vi "FTW-CodeGen-GetGrowInfo.vi"(0 "State In":T2, 5 "XRef":refnum<vi>) -> (1 "Spacing Between Terminals":i32=8 format="%d pixels", 2 "Timing Terminal Height":i32=8 format="%d pixels", 3 "Timing Terminals":i32[](array[numeric]) format="%d pixels", 4 "Grow Info":T1, 6 "Current Height":i32=8 format="%d pixels", 8 "Width":i32=8 format="%d pixels", 10 "Terminal Height":i32=8 format="%d pixels", 13 "Bottom Banner Height":i32=8 format="%d pixels", 14 "Total Top Banner Height":i32=8 format="%d pixels")   [LabVIEW 2014, in "FTW-Dataflow-Synchronizer.xnode"]
uses:
  FTW-Dataflow-Synchronizer.xnode
  FTW-CodeGen-State.ctl
panel:
  # "Inputs"
  # "Outputs"
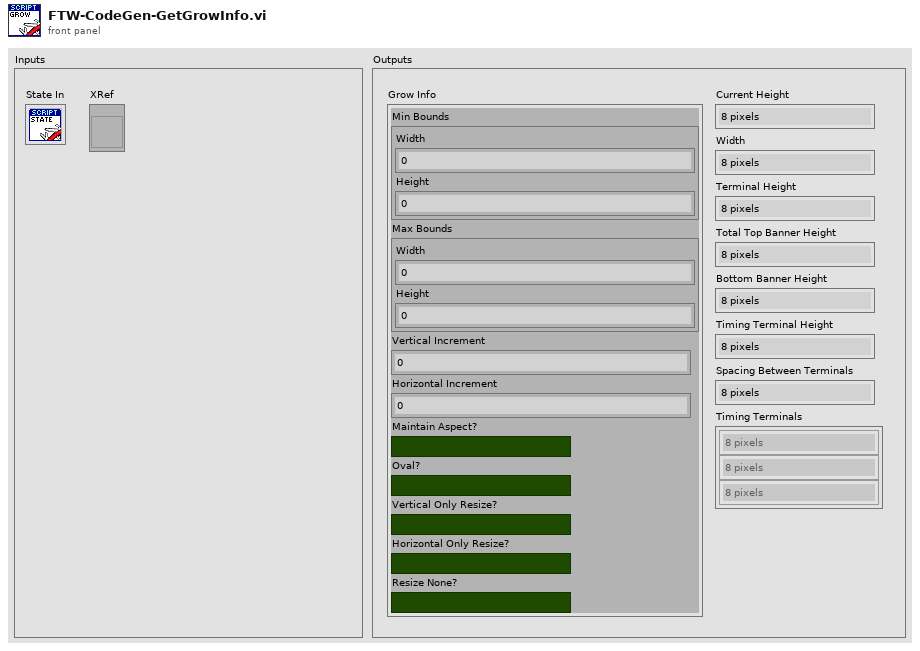
[diagram p1: front panel]
types:
  T1 = cluster{"Min Bounds":cluster{"Width":i32, "Height":i32}, "Max Bounds":cluster{"Width":i32, "Height":i32}, "Vertical Increment":i32, "Horizontal Increment":i32, "Maintain Aspect?":bool, "Oval?":bool, "Vertical Only Resize?":bool, "Horizontal Only Resize?":bool, "Resize None?":bool}
  T2 = typedef "FTW-Dataflow-Synchronizer.xnode/FTW-CodeGen-State.ctl" = cluster{"InputTerminals":cluster{"Wired?":bool, "ID":string, "DataName":string, "DataColor":u32, "Type":variant}[], "EnableTiming?":bool}
  T3 = cluster{"Wired?":bool, "ID":string, "DataName":string, "DataColor":u32, "Type":variant}[]
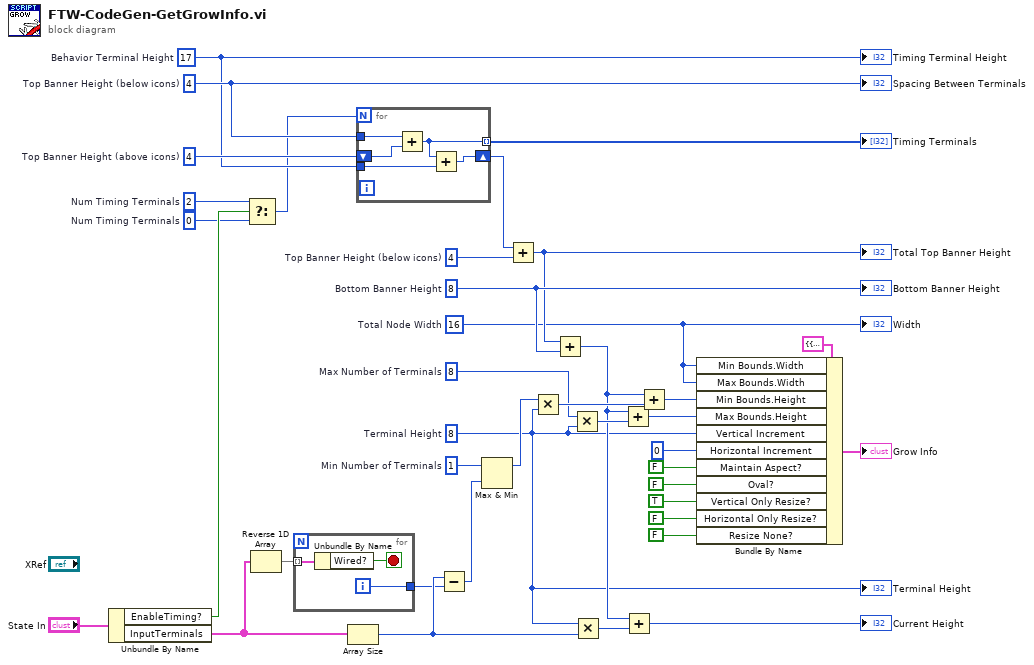
[diagram p0: block diagram]
diagram:
  w5 = 0  # Num Timing Terminals
  w7 = 2  # Num Timing Terminals
  w10 = 4  # Top Banner Height (below icons)
  w14 = 4  # Top Banner Height (below icons)
  w9 = 17  # Behavior Terminal Height
  w2 = 8  # Terminal Height
  w26 = 8  # Max Number of Terminals
  w21 = 8  # Bottom Banner Height
  w13 = 4  # Top Banner Height (above icons)
  w20 = 1  # Min Number of Terminals
  w1 = 16  # Total Node Width
  n1 = Unbundle By Name("State In") -> ("EnableTiming?"=w8:bool, "InputTerminals"=w4:T3)
  n2 = Select(t=w7, s=w8, f=w5) -> (s? t:f=w6:i32)
  n3 = Reverse 1D Array(array=w4) -> (reversed array=w18:T3)
  n4 = for {
    tunnel: w18 -> [w41] mode=indexing
    tunnel: [w40] -> w16
    i -> [w40]
    stop <- w39 stop-if-true
    n5 = Unbundle By Name(w41) -> ("Wired?"=w39:bool)
  }
  n6 = Array Size(array=w4) -> (size(s)=w17:i32)
  n7 = for {
    N: w6 -> [_]
    shift-right: [w45] -> w12
    shift-left: w13 -> [w46]
    tunnel: w9 -> [w44]
    tunnel: [w43] -> w11 mode=indexing
    tunnel: w10 -> [w42]
    n8 = Add(x=w42, y=w46) -> (x+y=w43:i32)
    n9 = Add(x=w43, y=w44) -> (x+y=w45:i32)
  }
  "Timing Terminals" <- w11
  n10 = Subtract(x=w17, y=w16) -> (x-y=w15:i32)
  n11 = Max & Min(x=w20, y=w15) -> (max(x,y)=w19:i32)  [unwired: 1 out]
  n12 = Add(x=w12, y=w14) -> (x+y=w3:i32)
  "Total Top Banner Height" <- w3
  n13 = Multiply(x=w19, y=w2) -> (x*y=w28:i32)
  n14 = Add(x=w3, y=w21) -> (x+y=w23:i32)
  n15 = Multiply(x=w26, y=w2) -> (x*y=w27:i32)
  n16 = Multiply(x=w2, y=w17) -> (x*y=w24:i32)
  n17 = Add(x=w23, y=w27) -> (x+y=w29:i32)
  n18 = Add(x=w23, y=w24) -> (x+y=→"Current Height":i32)
  n19 = Add(x=w23, y=w28) -> (x+y=w30:i32)
  n20 = Bundle By Name(cluster=T1 {"Min Bounds"={"Width"=0, "Height"=0}, "Max Bounds"={"Width"=0, "Height"=0}, "Vertical Increment"=0, "Horizontal Increment"=0, "Maintain Aspect?"=FALSE, "Oval?"=FALSE, "Vertical Only Resize?"=FALSE, "Horizontal Only Resize?"=FALSE, "Resize None?"=FALSE} ("Grow Info"), "Min Bounds.Width"=w1, "Max Bounds.Width"=w1, "Min Bounds.Height"=w30, "Max Bounds.Height"=w29, "Vertical Increment"=w2, "Horizontal Increment"=0, "Maintain Aspect?"=FALSE, "Oval?"=FALSE, "Vertical Only Resize?"=TRUE, "Horizontal Only Resize?"=FALSE, "Resize None?"=FALSE) -> (→"Grow Info":T1)
  "Terminal Height" <- w2
  "Width" <- w1
  "Bottom Banner Height" <- w21
  "Timing Terminal Height" <- w9
  "Spacing Between Terminals" <- w10
